vi "Plot StripLeadingDelim.vi"(11 "Start String":string) -> (1 "Error":bool, 2 "Remaining String":string, 3 "Delim":string)   [LabVIEW 2020, in "3D Plot.lvclass"]
uses:
  <vilib>/Math Plots/3D Math Plots/3D Plot/3D Plot/3D Plot.lvclass
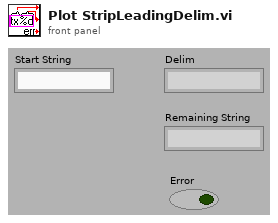
[diagram p1: front panel]
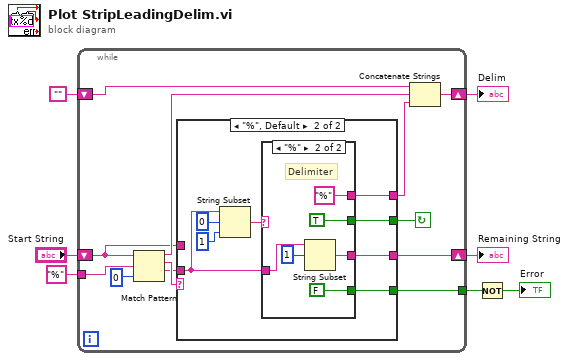
[diagram p0: block diagram]
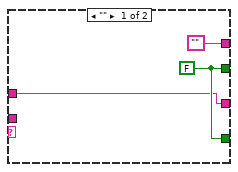
[diagram p2: hidden frame]
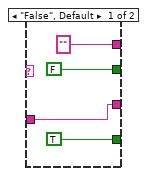
[diagram p3: hidden frame]
diagram:
  n1 = while {
    tunnel: "%" ("regular expression") -> [w19]
    shift-right: [w17] -> w5
    shift-left: "" -> [w18]
    tunnel: [w13] -> w6
    shift-right: [w9] -> w7
    shift-left: "Start String" -> [w8]
    stop <- w14 continue-if-true
    n2 = Match Pattern(string=w8, regular expression=w19, offset (0)=0) -> (before substring=w16:string, match substring=w11:string, after substring=w10:string)  [unwired: 1 out]
    n3 = case shown="\"%\", Default" w11 {
      tunnel: ["" w27] -> w15
      tunnel: [w21 w26] -> w14
      tunnel: [w21 w25] -> w13
      tunnel: w10 -> [_ w24]
      tunnel: [w20 w23] -> w9
      tunnel: w8 -> [w20 _]
      frame "" {
        w21 = FALSE
      }
      frame "%", Default {
        n4 = String Subset(string=w24, offset (0)=0, length (rest)=1 ("length (rest)")) -> (substring=w28:string)
        n5 = case shown="\"%\"" w28 {
          tunnel: ["" "%"] -> w27
          tunnel: [FALSE TRUE] -> w26
          tunnel: [TRUE FALSE] -> w25
          tunnel: w24 -> [w31 w37]
          tunnel: [w31 w35] -> w23
          frame "False", Default {
          }
          frame "%" {
            # "Delimiter"
            n6 = String Subset(string=w37, offset (0)=1) -> (substring=w35:string)  [unwired: 1 out]
          }
        }
      }
    }
    n7 = Concatenate Strings(w18, w16, w15) -> (w17:string)
  }
  "Remaining String" <- w7
  "Delim" <- w5
  n8 = Not(x=w6) -> (.not. x?=→"Error":bool)
